vi "Unit Test.vi"() -> ()   [LabVIEW 2018, in "Configuration File.lvlib" / "Configuration File.lvclass"]
doc: "This VI was built to test our config file system."
uses:
  Configuration File.lvclass
  <vilib>/Utility/config.llb/Write Key (String).vi
  <vilib>/Utility/config.llb/NI_LVConfig.lvlib
panel:
  in  "name or relative path":string="ConfigFileSettings.ini"
  out "Pass?":bool
  out "error out":errorcluster
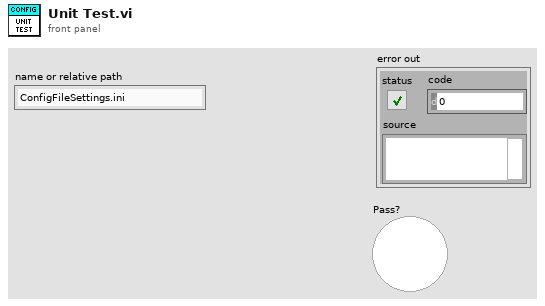
[diagram p1: front panel]
types:
  T1 = typedef "NI_LVConfig.lvlib/Config Data RefNum.ctl" = refnum<k1>
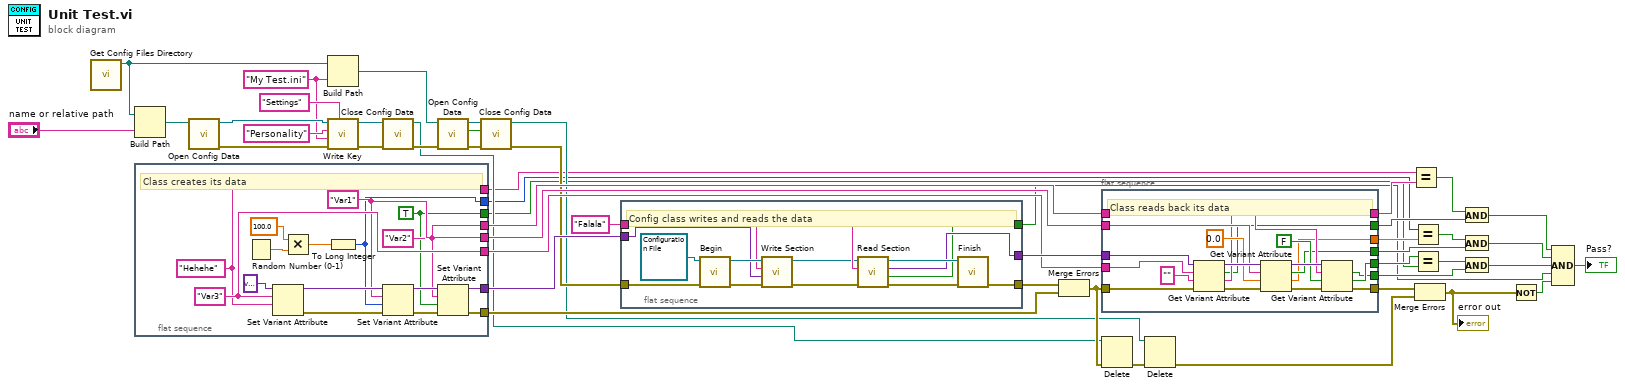
[diagram p0: block diagram]
diagram:
  w20 = "My Test.ini" ("name or relative path")
  n1 = call "Get Config Files Directory.vi"() -> ("configuration file path"=w23:path)  [unwired: 11 in]
  n2 = Build Path(base path=w23, name or relative path="name or relative path") -> (appended path=w21:path)
  n3 = flat-sequence {
    tunnel: [w60] -> w49
    tunnel: [w59] -> w46
    tunnel: [w58] -> w45
    tunnel: [w57] -> w44
    tunnel: [w56] -> w43
    tunnel: [w55] -> w18
    tunnel: [w50] -> w3
    tunnel: [w53] -> w2
    frame #0 {
      w53 = TRUE
      w57 = "Var2" ("name")
      w58 = "Var1" ("name")
      w55 = "Hehehe"
      w59 = "Var3" ("name")
      # "Class creates its data"
      n4 = Random Number (0-1)() -> (number: 0 to 1=w54:dbl)
      n5 = Set Variant Attribute(Variant=variant, name=w59, value=w55) -> (Variant out=w64:variant, error out=w63:errorcluster)  [unwired: 1 in, 1 out]
      n6 = Multiply(x=100.0, y=w54) -> (x*y=w52:dbl)
      n7 = To Long Integer(number=w52) -> (32bit integer=w50:i32)
      n8 = Set Variant Attribute(Variant=w64, name=w58, value=w50, error in=w63) -> (Variant out=w62:variant, error out=w61:errorcluster)  [unwired: 1 out]
      n9 = Set Variant Attribute(Variant=w62, name=w57, value=w53, error in=w61) -> (Variant out=w60:variant, error out=w56:errorcluster)  [unwired: 1 out]
    }
  }
  n10 = call <vilib>:"Open Config Data.vi"("configuration file path"=w21) -> ("error out"=w40:errorcluster, "refnum"=w41:T1)  [unwired: 8 in, 1 out]
  n11 = Build Path(base path=w23, name or relative path=w20) -> (appended path=w24:path)
  n12 = call-poly <vilib>:"Write Key.vi"("section"="Settings", "error in (no error)"=w40, "value"=w20, "key"="Personality", "refnum"=w41) -> ("error out"=w38:errorcluster, "refnum out"=w39:T1)  [unwired: 4 in, 1 out]
  n13 = call <vilib>:"Close Config Data.vi"("error in (no error)"=w38, "refnum"=w39) -> ("error out"=w37:errorcluster, "file path"=w27:path)  [unwired: 8 in]
  n14 = call <vilib>:"Open Config Data.vi"("error in (no error)"=w37, "configuration file path"=w24) -> ("error out"=w31:errorcluster, "file created?"=w30:bool, "refnum"=w32:T1)  [unwired: 7 in]
  n15 = call <vilib>:"Close Config Data.vi"("error in (no error)"=w31, "write file if changed (T)"=w30, "refnum"=w32) -> ("error out"=w29:errorcluster, "file path"=w28:path)  [unwired: 7 in]
  n16 = flat-sequence {
    tunnel: w49 -> [w73]
    tunnel: "Falala" ("Section Name") -> [w72]
    tunnel: [w71] -> w47
    tunnel: [w68] -> w42
    tunnel: w29 -> [w67]
    tunnel: [w66] -> w6
    frame #0 {
      # "Config class writes and reads the data"
      n17 = call-dynamic "Begin.vi"("error in (no error)"=w67, "Configuration File in"=refnum<class "Configuration File.lvclass"> refnum ("Configuration File.lvlib:Configuration File.lvclass")) -> ("error out"=w77:errorcluster, "Configuration File out"=w78:refnum<class "Configuration File.lvclass">)  [unwired: 8 in]
      n18 = call-dynamic "Write Section.vi"("error in (no error)"=w77, "Section Data"=w73, "Section Name"=w72, "Configuration File in"=w78) -> ("error out"=w76:errorcluster, "Configuration File out"=w69:refnum<class "Configuration File.lvclass">)  [unwired: 6 in]
      n19 = call-dynamic "Read Section.vi"("error in (no error)"=w76, "Section Name"=w72, "Configuration File in"=w69) -> ("error out"=w70:errorcluster, "Found section and keys?"=w66:bool, "Data Out"=w71:variant, "Configuration File out"=w75:refnum<class "Configuration File.lvclass">)  [unwired: 5 in]
      n20 = call-dynamic "Finish.vi"("error in (no error)"=w70, "Configuration File in"=w75) -> ("error out"=w68:errorcluster)  [unwired: 6 in, 3 out]
    }
  }
  n21 = Merge Errors(w42, w43) -> (w36:errorcluster)
  n22 = flat-sequence {
    tunnel: w47 -> [w97]
    tunnel: w46 -> [w92]
    tunnel: w45 -> [w91]
    tunnel: w44 -> [w90]
    tunnel: [w86] -> w12
    tunnel: [w85] -> w11
    tunnel: w36 -> [w84]
    tunnel: [w83] -> w34
    tunnel: [w82] -> w19
    tunnel: [w81] -> w16
    tunnel: [w80] -> w10
    tunnel: [w79] -> w9
    frame #0 {
      # "Class reads back its data"
      n23 = Get Variant Attribute(Variant=w97, name=w92, default value (empty Variant)="", error in=w84) -> (duplicate Variant=w96:variant, found=w81:bool, value=w82:string, error out=w94:errorcluster)
      n24 = Get Variant Attribute(Variant=w96, name=w91, default value (empty Variant)=0.0, error in=w94) -> (duplicate Variant=w95:variant, found=w80:bool, value=w79:dbl, error out=w93:errorcluster)
      n25 = Get Variant Attribute(Variant=w95, name=w90, default value (empty Variant)=FALSE, error in=w93) -> (found=w85:bool, value=w86:bool, error out=w83:errorcluster)  [unwired: 1 out]
    }
  }
  n26 = Delete(path (use dialog)=w27, error in=w36) -> (error out=w35:errorcluster)  [unwired: 3 in, 2 out]
  n27 = Delete(path (use dialog)=w28, error in=w35) -> (error out=w33:errorcluster)  [unwired: 3 in, 2 out]
  n28 = Equal?(x=w18, y=w19) -> (x = y?=w17:bool)
  n29 = Equal?(x=w3, y=w9) -> (x = y?=w14:bool)
  n30 = Equal?(x=w12, y=w2) -> (x = y?=w13:bool)
  n31 = Merge Errors(w34, w33) -> (w5:errorcluster)
  "error out" <- w5
  n32 = And(x=w17, y=w16) -> (x .and. y?=w15:bool)
  n33 = And(x=w14, y=w10) -> (x .and. y?=w8:bool)
  n34 = And(x=w13, y=w11) -> (x .and. y?=w7:bool)
  n35 = Not(x=w5) -> (.not. x?=w4:bool)
  n36 = Compound Arithmetic op=AND(w15, w8, w7, w6, w4) -> (→"Pass?":bool)
